vi "Calculator.vi"() -> ()   [LabVIEW 2015]
panel:
  in  "Answer Color":u32(colorbox)
  in  "Enum":T1(ring)
  in  "B":dbl
  in  "A":dbl
  out "Answer":u32 format="%.0x"
  # "Calculator"
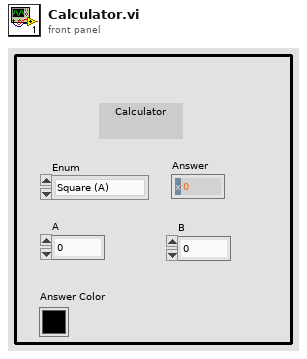
[diagram p1: front panel]
types:
  T1 = enum32{"Square (A)", "Add", "Subtract", "Multiply", "Divide"}
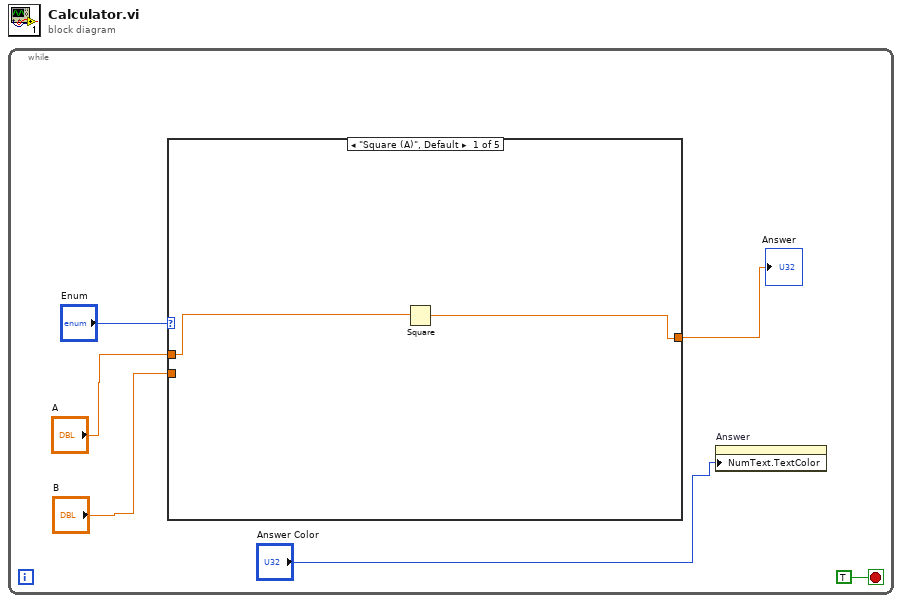
[diagram p0: block diagram]
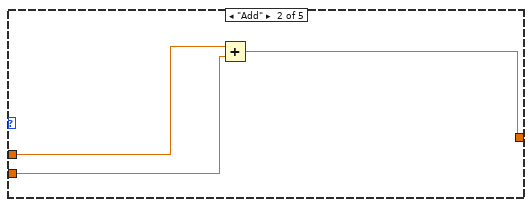
[diagram p2: hidden frame]
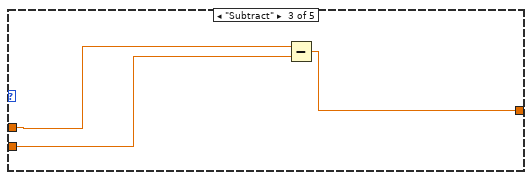
[diagram p3: hidden frame]
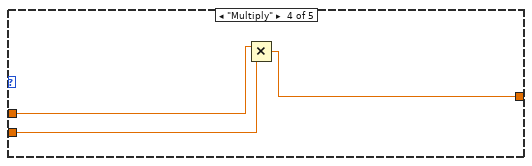
[diagram p4: hidden frame]
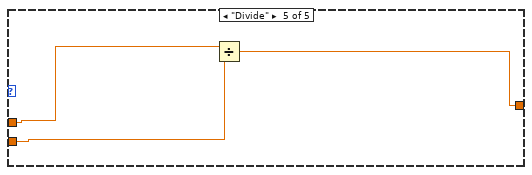
[diagram p5: hidden frame]
diagram:
  n1 = while {
    stop <- TRUE stop-if-true
    n2 = case shown="\"Square (A)\", Default" "Enum" {
      tunnel: [w8 w11 w12 w15 w20] -> w3
      tunnel: "A" -> [w7 w10 w13 w17 w18]
      tunnel: "B" -> [_ w9 w14 w16 w19]
      frame "Square (A)", Default {
        n3 = Square(x=w7) -> (x^2=w8:dbl)
      }
      frame "Add" {
        n4 = Add(x=w10, y=w9) -> (x+y=w11:dbl)
      }
      frame "Subtract" {
        n5 = Subtract(x=w13, y=w14) -> (x-y=w12:dbl)
      }
      frame "Multiply" {
        n6 = Multiply(x=w17, y=w16) -> (x*y=w15:dbl)
      }
      frame "Divide" {
        n7 = Divide(x=w18, y=w19) -> (x/y=w20:dbl)
      }
    }
    "Answer" <- w3
    n8 = property on="Answer" class="DigNum (strict)"("NumText.TextColor"="Answer Color") -> ()  [unwired: 2 in, 2 out]
  }
